vi "SVPO Envelope Detection (N Ch DBL Array).vi"(0 "scaled signals [EU]":dbl[][](array[numeric]), 1 "reset? (F)":bool, 5 "sampling rate [Hz]":dbl=1.0, 9 "band specification":T1={"center frequency [Hz]"=4800.0, "span [Hz]"=2000.0}) -> (4 "envelope signals [EU]":dbl[][](array[numeric]), 6 "sampling rate out [Hz]":dbl)   [LabVIEW 2017, in "SoundVib_FaultAnalysis.lvlib"]
doc: "Extracts the modulating signal, or envelope signal, from an amplitude-modulated signal. You can use the envelope detection technique to identify the mechanical faults that have amplitude-modulating effect on the vibration signal of a machine. Use this VI on embedded targets that have limited computational resources. Wire data to the <B>scaled signal [EU]</B> input to determine the polymorphic instance to use or manually select the instance."
uses:
  <vilib>/addons/Sound and Vibration/Order Analysis/Fault Analysis/SoundVib_FaultAnalysis.lvlib
  <vilib>/addons/Sound and Vibration/Order Analysis/Resample Order Tracking/SubVIs/oa_Calculate CIC Decimation Filter Coefficients.vi
  <vilib>/addons/Sound and Vibration/Order Analysis/Fault Analysis/SubVIs/sv_Compute Shift and Low Pass Filter with IC.vi
  <vilib>/addons/Sound and Vibration/Order Analysis/Resample Order Tracking/SubVIs/OAT Frequency Shift (Mixer).vi
  <vilib>/addons/Sound and Vibration/Order Analysis/Resample Order Tracking/SubVIs/oa_Decimation with CIC and Compensation Filter.vi
  <vilib>/addons/Sound and Vibration/Order Analysis/Fault Analysis/SubVIs/oa_Demodulation Initial States (1 Channel).vi
  <vilib>/addons/Sound and Vibration/Order Analysis/Adv Resampling/OAT Single Stage Decimation with IC.vi
  <vilib>/addons/Sound and Vibration/Order Analysis/Resample Order Tracking/SubVIs/OAT CIC Decimation.vi
  <vilib>/addons/Sound and Vibration/Order Analysis/Resample Order Tracking/SubVIs/oa_Interpolate Zeros Between Samples.vi
  <vilib>/addons/Sound and Vibration/Order Analysis/Resample Order Tracking/SubVIs/oa_Calculate Delay of CIC Decimation Interpolation Filter.vi
  <vilib>/addons/Sound and Vibration/Order Analysis/Resample Order Tracking/SubVIs/oa_Create CIC Compensation Filter.vi
  <vilib>/addons/Sound and Vibration/Order Analysis/Resample Order Tracking/SubVIs/oa_Create CIC LP Truncation Filter.vi
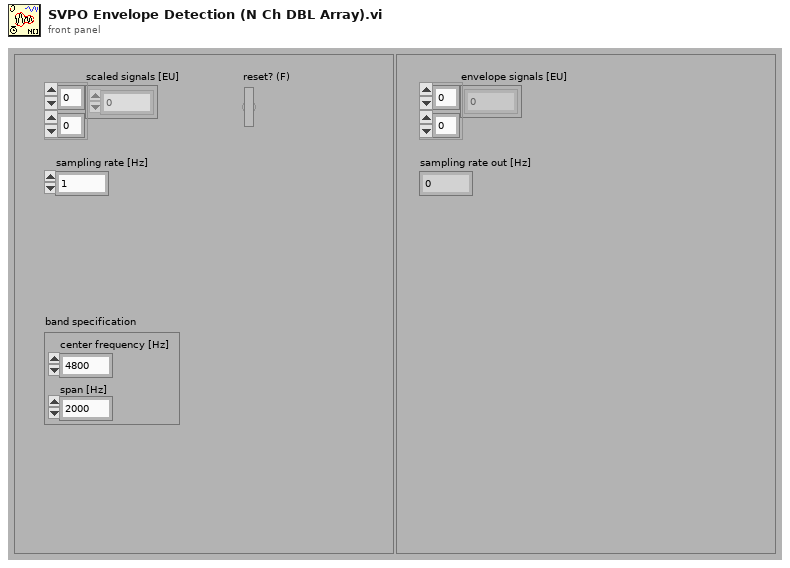
[diagram p1: front panel]
types:
  T1 = cluster{"center frequency [Hz]":dbl, "span [Hz]":dbl}
  T2 = typedef "OAT Decimation Filter.ctl" = cluster{"coefficients":dbl[], "factor":i32}
  T3 = cluster{"filter settings":cluster{"CIC Settings":cluster{"Numeric":i32, i32, i32}, "filters":T2[], "delay":i32, "interpolation factor":i32}, "filter states":cluster{"t0":dbl, "phase":dbl, "real filter state":cluster{cluster{dbl[]}, cluster{dbl[]}[]}, "imaginary filter state":cluster{cluster{dbl[]}, cluster{dbl[]}[]}, "delay":i32}[], "reset pending":bool}
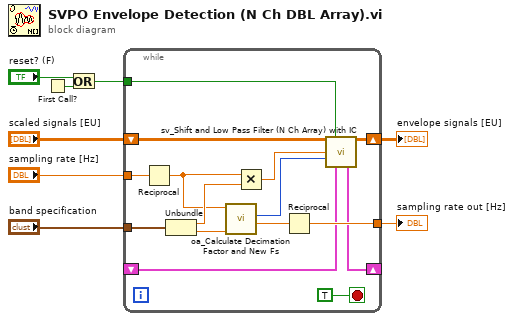
[diagram p0: block diagram]
diagram:
  n1 = First Call?() -> (First Call?: T/F=w6:bool)
  n2 = Or(x="reset? (F)", y=w6) -> (x .or. y?=w5:bool)
  n3 = while {
    tunnel: "band specification" -> [w23]
    tunnel: w5 -> [w18]
    tunnel: "sampling rate [Hz]" -> [w17]
    tunnel: [w12] -> w1
    shift-right: [w10] -> _
    shift-left: _ -> [w9]
    shift-right: [w14] -> w2
    shift-left: "scaled signals [EU]" -> [w15]
    stop <- TRUE stop-if-true
    n4 = Reciprocal(x=w17) -> (1/x=w16:dbl)
    n5 = Unbundle(w23) -> ("center frequency [Hz]"=w19:dbl, "span [Hz]"=w20:dbl)
    n6 = call <vilib>:"oa_Calculate Decimation Factor and New Fs.vi"("span"=w20, "dt"=w16) -> ("new dt"=w13:dbl, "decimation factor"=w22:i32)  [unwired: 8 in]
    n7 = Multiply(x=w16, y=w19) -> (x*y=w21:dbl)
    n8 = Reciprocal(x=w13) -> (1/x=w12:dbl)
    n9 = call <vilib>:"sv_Shift and Low Pass Filter (N Ch Array) with IC.vi"("input signals"=w15, "reset? (F)"=w18, "center"=w21, "decimation factor"=w22, "initial conditions"=w9) -> ("enveloped signals"=w14:dbl[][], "final conditions"=w10:T3)  [unwired: 7 in, 2 out]
  }
  "sampling rate out [Hz]" <- w1
  "envelope signals [EU]" <- w2
